vi "Create V Chans_RTM.vi"(6 "Remote Sense?":T1, 7 "Device Ref in":T2 format="%.0x", 8 "error in":errorcluster, 9 "Channels to Add":u16[](array[numeric]), 10 "Current Limit":dbl, 11 "Init Value":dbl) -> (0 "error out":errorcluster)   [LabVIEW 2018, in "NI PXI-4110 Programmable Power Supply Custom Device.lvlib"]
uses:
  NI PXI-4110 Programmable Power Supply Custom Device.lvlib
  <vilib>/NI Veristand/Custom Device API/Custom Device Item Ref.ctl
  RemoteSense.ctl
  <vilib>/NI Veristand/Custom Device API/Custom Device Channel.ctl
  <vilib>/NI Veristand/Custom Device API/Custom Device Channel Type.ctl
  4110_Global.vi
  <vilib>/NI Veristand/Custom Device API/Get Item Property (U16).vi
  <vilib>/NI Veristand/Custom Device API/Set Item Property (U16).vi
  <vilib>/NI VeriStand/Custom Device API/Custom Device API.lvlib
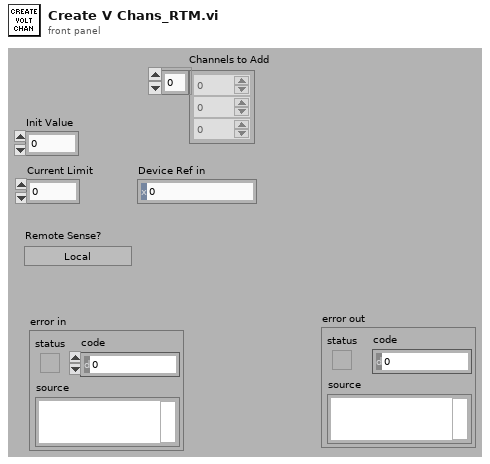
[diagram p1: front panel]
types:
  T1 = typedef "NI PXI-4110 Programmable Power Supply Custom Device.lvlib/RemoteSense.ctl" = bool
  T2 = typedef "Custom Device API.lvlib/Custom Device Item Ref.ctl" = u64
  T3 = typedef "Custom Device API.lvlib/Custom Device Channel.ctl" = cluster{"Type":T4, "Units":string, "Default Value":dbl, "Faultable":bool, "Scalable":bool}
  T4 = typedef "Custom Device API.lvlib/Custom Device Channel Type.ctl" = enum16{"Input", "Output"}
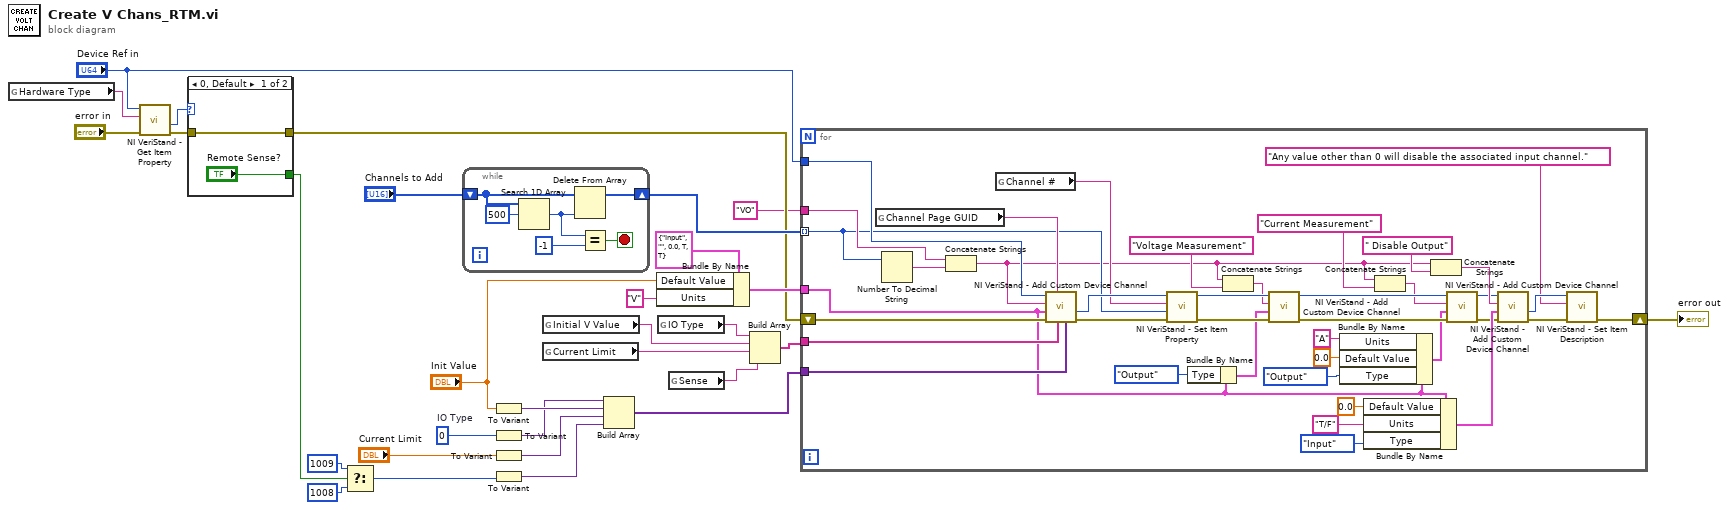
[diagram p0: block diagram]
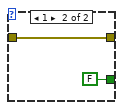
[diagram p2: hidden frame]
diagram:
  w19 = u16 0  # IO Type
  n1 = global read "4110_Global.vi" "Hardware Type"() -> (w12:string)
  n2 = call-poly <vilib>:"NI VeriStand - Get Item Property.vi"("error in (no error)"="error in", "Property Name"=w12, "Item Ref in"="Device Ref in") -> ("error out"=w9:errorcluster, "Value"=w10:u16)  [unwired: 5 in, 2 out]
  n3 = case shown="0, Default" w10 {
    tunnel: w9 -> [w32 w34]
    tunnel: [w32 w34] -> w8
    tunnel: ["Remote Sense?" T1 FALSE ("Remote Sense?")] -> w5
    frame 0, Default {
    }
    frame 1 {
    }
  }
  n4 = Select(t=1009, s=w5, f=1008) -> (s? t:f=w2:i32)
  n5 = while {
    shift-right: [w36] -> w14
    shift-left: "Channels to Add" -> [w37]
    stop <- w35 stop-if-true
    n6 = Search 1D Array(1D array=w37, element=u16 500) -> (index of element=w39:i32)  [unwired: 1 in]
    n7 = Delete From Array(array=w37, index=w39) -> (array with subset deleted=w36:u16[])  [unwired: 1 in, 1 out]
    n8 = Equal?(x=w39, y=-1) -> (x = y?=w35:bool)
  }
  n9 = To Variant(anything="Init Value") -> (Variant=w27:variant)
  n10 = To Variant(anything=w19) -> (Variant=w26:variant)
  n11 = To Variant(anything="Current Limit") -> (Variant=w28:variant)
  n12 = To Variant(anything=w2) -> (Variant=w6:variant)
  n13 = global read "4110_Global.vi" "Initial V Value"() -> (w21:string)
  n14 = global read "4110_Global.vi" "Current Limit"() -> (w20:string)
  n15 = Build Array(w26, w27, w28, w6) -> (w29:variant[])
  n16 = Bundle By Name(cluster=T3 {"Type"=enum."Input", "Units"="", "Default Value"=0.0, "Faultable"=TRUE, "Scalable"=TRUE} ("Channel"), "Default Value"="Init Value", "Units"="V") -> (w23:T3)
  n17 = global read "4110_Global.vi" "IO Type"() -> (w22:string)
  n18 = global read "4110_Global.vi" "Sense"() -> (w7:string)
  n19 = Build Array(w22, w21, w20, w7) -> (w30:string[])
  n20 = for {
    shift-right: [w55] -> w25
    shift-left: w8 -> [w79]
    tunnel: w23 -> [w46]
    tunnel: "Device Ref in" -> [w78]
    tunnel: "VO" ("string") -> [w77]
    tunnel: w29 -> [w73]
    tunnel: w30 -> [w72]
    tunnel: w14 -> [w69] mode=indexing
    n21 = global read "4110_Global.vi" "Channel Page GUID"() -> (w70:string)
    n22 = Number To Decimal String(number=w69) -> (decimal integer string=w76:string)  [unwired: 1 in]
    n23 = Concatenate Strings(w77, w76) -> (w49:string)
    n24 = global read "4110_Global.vi" "Channel #"() -> (w71:string)
    n25 = call <vilib>:"NI VeriStand - Add Custom Device Channel.vi"("Property Values"=w73, "Property names"=w72, "GUID (Default Channel)"=w70, "error in (no error)"=w79, "Channel"=w46, "Channel Name"=w49, "Parent Ref in"=w78) -> ("error out"=w75:errorcluster, "Channel Ref"=w74:T2)  [unwired: 1 in, 2 out]
    n26 = call-poly <vilib>:"NI VeriStand - Set Item Property.vi"("error in (no error)"=w75, "Value"=w69, "Property Name"=w71, "Item Ref in"=w74) -> ("error out"=w68:errorcluster, "Item Ref out"=w67:T2)  [unwired: 5 in, 1 out]
    n27 = Bundle By Name(cluster=w46, "Type"=Custom_Device_Channel_Type."Output") -> (w63:T3)
    n28 = Concatenate Strings(w49, "Voltage Measurement" ("string")) -> (w65:string)
    n29 = call <vilib>:"NI VeriStand - Add Custom Device Channel.vi"("error in (no error)"=w68, "Channel"=w63, "Channel Name"=w65, "Parent Ref in"=w67) -> ("error out"=w51:errorcluster, "Parent Ref out"=w52:T2)  [unwired: 4 in, 2 out]
    n30 = Bundle By Name(cluster=w46, "Units"="A", "Default Value"=0.0, "Type"=Custom_Device_Channel_Type."Output") -> (w43:T3)
    n31 = Bundle By Name(cluster=w46, "Default Value"=0.0, "Units"="T/F", "Type"=Custom_Device_Channel_Type."Input") -> (w57:T3)
    n32 = Concatenate Strings(w49, "Current Measurement" ("string")) -> (w48:string)
    n33 = Concatenate Strings(w49, " Disable Output" ("string")) -> (w61:string)
    n34 = call <vilib>:"NI VeriStand - Add Custom Device Channel.vi"("error in (no error)"=w51, "Channel"=w43, "Channel Name"=w48, "Parent Ref in"=w52) -> ("error out"=w41:errorcluster, "Parent Ref out"=w42:T2)  [unwired: 4 in, 2 out]
    n35 = call <vilib>:"NI VeriStand - Add Custom Device Channel.vi"("error in (no error)"=w41, "Channel"=w57, "Channel Name"=w61, "Parent Ref in"=w42) -> ("error out"=w56:errorcluster, "Channel Ref"=w54:T2)  [unwired: 4 in, 2 out]
    n36 = call <vilib>:"NI VeriStand - Set Item Description.vi"("error in (no error)"=w56, "Description"="Any value other than 0 will disable the associated input channel.", "Item Ref in"=w54) -> ("error out"=w55:errorcluster)  [unwired: 6 in, 2 out]
  }
  "error out" <- w25
